vi "ConfigureSyringeBD.vi"(0 "object in":refnum<class "CetoniPump.lvclass">, 1 "index":i32, 2 "Syringe":T1(ring), 5 "error in (no error)":errorcluster) -> (14 "object out":refnum<class "CetoniPump.lvclass">, 19 "error out":errorcluster)   [LabVIEW 2023, in "CetoniPump.lvclass"]
uses:
  CetoniPump.lvclass
panel:
  out "x*y":dbl
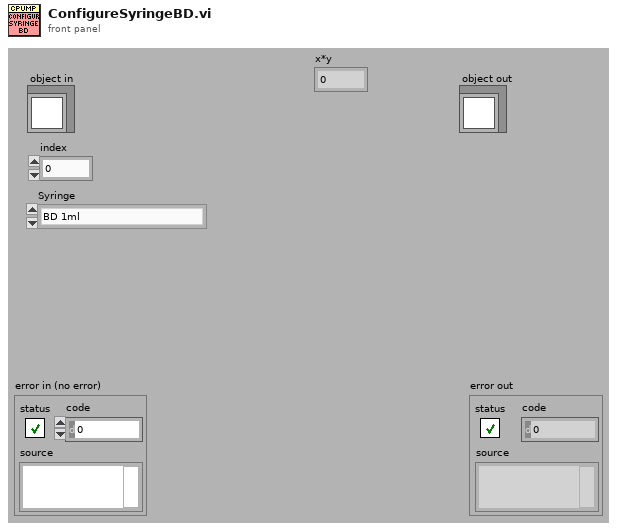
[diagram p1: front panel]
types:
  T1 = enum16{"BD 1ml", "BD 3ml", "BD 5ml", "BD 10ml", "BD 20ml", "BD 30ml", "BD 50ml", "HSW 1ml"}
  T2 = cluster{"Maximum Piston Stroke (mm)":dbl, "Inner Diameter (mm)":dbl}
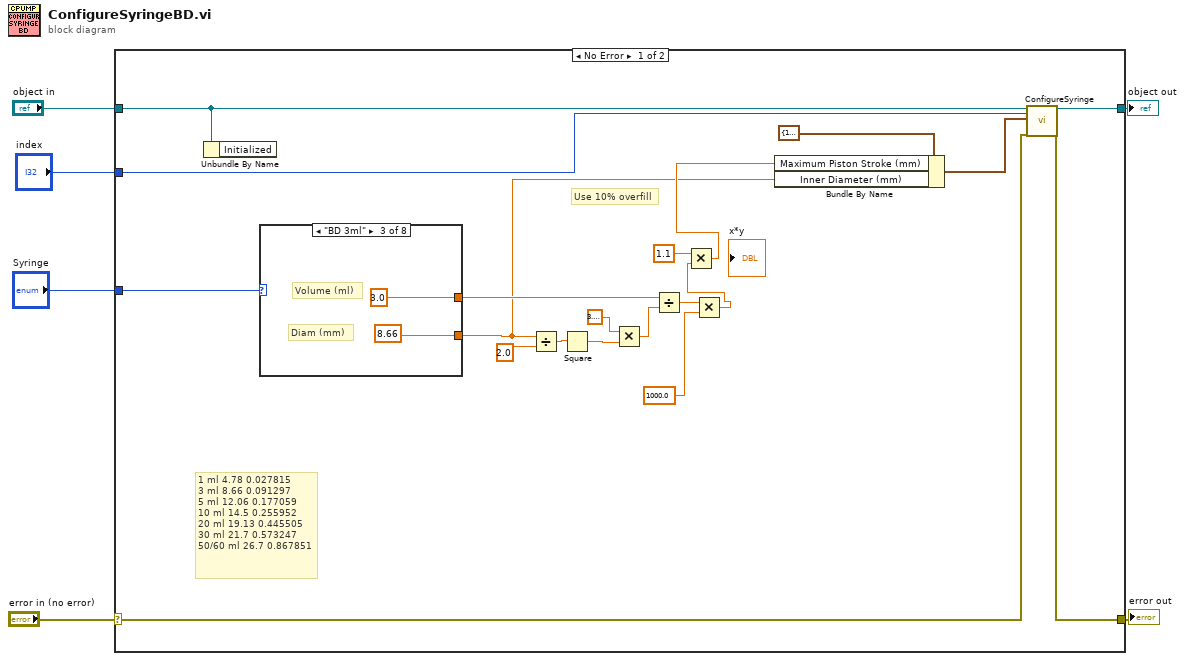
[diagram p0: block diagram]
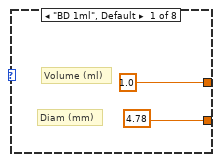
[diagram p2: hidden frame]
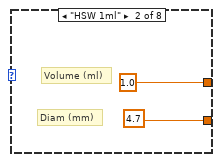
[diagram p3: hidden frame]
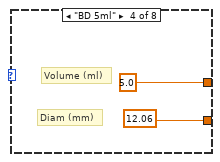
[diagram p4: hidden frame]
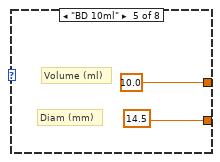
[diagram p5: hidden frame]
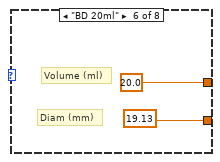
[diagram p6: hidden frame]
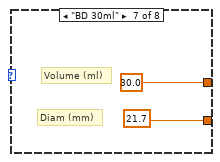
[diagram p7: hidden frame]
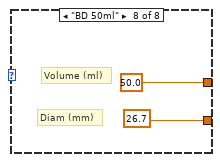
[diagram p8: hidden frame]
diagram:
  n1 = case shown="No Error" "error in (no error)" {
    selector: "error in (no error)" -> [w10 w44]
    tunnel: [w9 w44] -> w5
    tunnel: [w15 w43] -> w3
    tunnel: "object in" -> [w26 w43]
    tunnel: "index" -> [w8 _]
    tunnel: "Syringe" -> [w7 _]
    frame No Error {
      # "Use 10% overfill"
      # "1 ml 4.78 0.027815\n3 ml 8.66 0.091297\n5 ml 12.06 0.177059\n10 ml 14.5 0.255952\n20 ml 19.13 0.445505\n30 ml 21.7 0.573247\n50/60 ml 26.7 0.867851"
      n2 = Unbundle By Name(w26) -> ()  [unwired: 1 out]
      n3 = case shown="\"BD 3ml\"" w7 {
        tunnel: [1.0 1.0 3.0 5.0 10.0 20.0 30.0 50.0] -> w19
        tunnel: [4.78 4.7 8.66 12.06 14.5 19.13 21.7 26.7] -> w12
        frame "BD 1ml", Default {
          # "Diam (mm)"
          # "Volume (ml)"
        }
        frame "HSW 1ml" {
          # "Diam (mm)"
          # "Volume (ml)"
        }
        frame "BD 3ml" {
          # "Diam (mm)"
          # "Volume (ml)"
        }
        frame "BD 5ml" {
          # "Diam (mm)"
          # "Volume (ml)"
        }
        frame "BD 10ml" {
          # "Diam (mm)"
          # "Volume (ml)"
        }
        frame "BD 20ml" {
          # "Diam (mm)"
          # "Volume (ml)"
        }
        frame "BD 30ml" {
          # "Diam (mm)"
          # "Volume (ml)"
        }
        frame "BD 50ml" {
          # "Diam (mm)"
          # "Volume (ml)"
        }
      }
      n4 = Divide(x=w12, y=2.0) -> (x/y=w24:dbl)
      n5 = Square(x=w24) -> (x^2=w23:dbl)
      n6 = Multiply(x=3.141592653589793, y=w23) -> (x*y=w20:dbl)
      n7 = Divide(x=w19, y=w20) -> (x/y=w17:dbl)
      n8 = Multiply(x=w17, y=1000.0) -> (x*y=w16:dbl)
      n9 = Multiply(x=1.1, y=w16) -> (x*y=w13:dbl)
      n10 = Bundle By Name(cluster=T2 {"Maximum Piston Stroke (mm)"=100.0, "Inner Diameter (mm)"=12.0} ("SyringeSettings"), "Maximum Piston Stroke (mm)"=w13, "Inner Diameter (mm)"=w12) -> (w11:T2)
      n11 = call-dynamic "ConfigureSyringe.vi"("object in"=w26, "index"=w8, "SyringeSettings"=w11, "error in (no error)"=w10) -> ("object out"=w15:refnum<class "CetoniPump.lvclass">, "error out"=w9:errorcluster)  [unwired: 14 in]
    }
    frame Error {
    }
  }
  "error out" <- w5
  "object out" <- w3
